vi "BuildFileListFile.vi"(10 "Task":enum16{"BuildFile", "ReadFile"}(ring)=enum."ReadFile") -> (0 "error out":errorcluster, 3 "Instruments":cluster{"Folder Path":path, "tags":string[]}[](array[cluster]))   [LabVIEW 2022 SP3]
panel:
  out "text":string
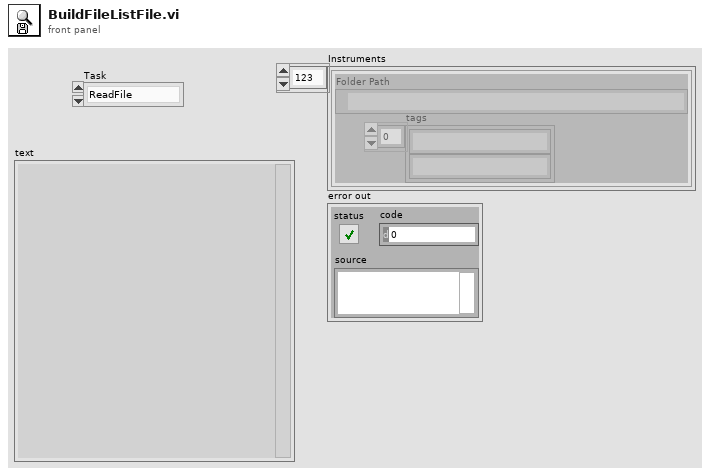
[diagram p1: front panel]
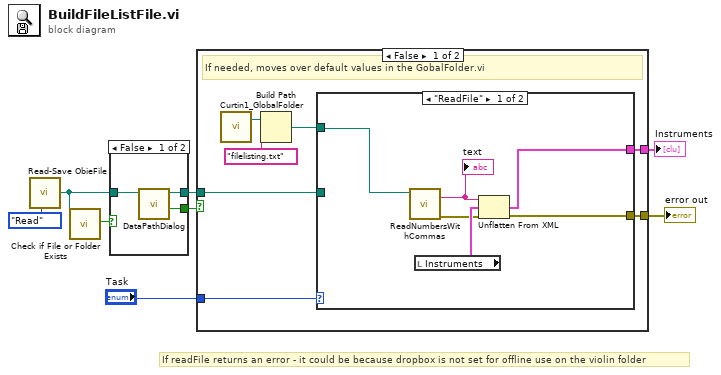
[diagram p0: block diagram]
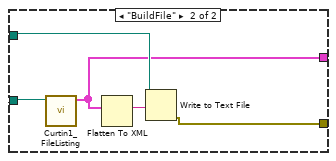
[diagram p2: hidden frame]
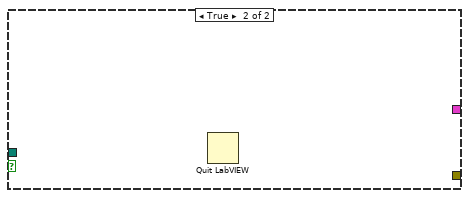
[diagram p3: hidden frame]
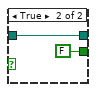
[diagram p4: hidden frame]
diagram:
  # "If readFile returns an error - it could be because dropbox is not set for offline use on the violin folder"
  n1 = call "Read-Save ObieFile.vi"("Task"=enum16{"Save", "Read"}."Read") -> ("DataPath Out"=w4:path)  [unwired: 8 in, 2 out]
  n2 = call <vilib>:"Check if File or Folder Exists.vi"("path"=w4) -> ("file or folder exists?"=w5:bool)  [unwired: 8 in, 2 out]
  n3 = case shown="False" w5 {
    tunnel: w4 -> [w11 w13]
    tunnel: [w10 w13] -> w2
    tunnel: [w9 FALSE ("canceled?")] -> w1
    frame False {
      n4 = call "DataPathDialog.vi"("Path"=w11) -> ("canceled?"=w9:bool, "Path out"=w10:path)  [unwired: 9 in]
    }
    frame True {
    }
  }
  n5 = case shown="False" w1 {
    tunnel: [w20 _] -> w8
    tunnel: "Task" -> [w19 _]
    tunnel: [w18 _] -> w6
    tunnel: w2 -> [w17 _]
    frame False {
      # "If needed, moves over default values in the GobalFolder.vi"
      n6 = call "Curtin1_GlobalFolder.vi"() -> ("LabVIEW Data Path"=w16:path)  [unwired: 1 in, 1 out]
      n7 = Build Path(base path=w16, name or relative path="filelisting.txt") -> (appended path=w14:path)
      n8 = case shown="\"ReadFile\"" w19 {
        tunnel: w14 -> [w23 w31]
        tunnel: [w26 w30] -> w20
        tunnel: [w24 w29] -> w18
        tunnel: w17 -> [_ w27]
        frame "ReadFile" {
          n9 = call "ReadNumbersWithCommas.vi"("file (use dialog)"=w23) -> ("error out"=w21:errorcluster, "text"=w22:string)  [unwired: 7 in, 2 out]
          "text" <- w22
          n10 = local read "Instruments"() -> (w25:cluster{"Folder Path":path, "tags":string[]}[])
          n11 = Unflatten From XML(xml string=w22, type=w25, error in (no error)=w21) -> (value=w24:cluster{"Folder Path":path, "tags":string[]}[], error out=w26:errorcluster)
        }
        frame "BuildFile" {
          n12 = call "Curtin1_FileListing.vi"("Folder Path"=w27) -> ("Array"=w29:cluster{"Folder Path":path, "tags":string[]}[])  [unwired: 10 in]
          n13 = Flatten To XML(6:w29) -> (2:w28:string)
          n14 = Write to Text File(file (use dialog)=w31, text=w28) -> (error out=w30:errorcluster)  [unwired: 2 in, 2 out]
        }
      }
    }
    frame True {
      n15 = Quit LabVIEW() -> ()  [unwired: 1 in]
    }
  }
  "error out" <- w8
  "Instruments" <- w6
